vi "open-islanding.vi"(7 "islanding config":T1={"GA-ip"="192.168.1.1", "write-port-ga"=32101, "listen-port"=32111, "res-ip"="127.0.0.1", "write-port-res"=32102}) -> (0 "error out":errorcluster, 5 "connection ID":refnum<k16>)   [LabVIEW 2021]
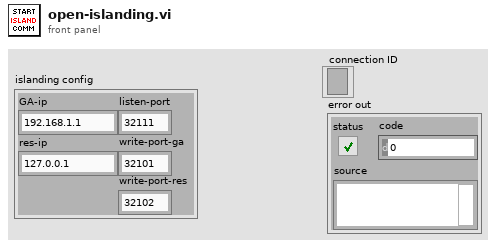
[diagram p1: front panel]
types:
  T1 = cluster{"GA-ip":string, "write-port-ga":u16, "listen-port":u16, "res-ip":string, "write-port-res":u16}
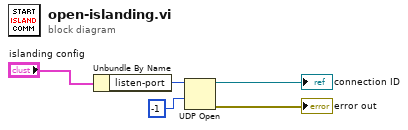
[diagram p0: block diagram]
diagram:
  n1 = Unbundle By Name("islanding config") -> ("listen-port"=w3:u16)
  n2 = UDP Open(9:-1 ("timeout ms (25000)"), 11:w3) -> (port=→"connection ID":refnum<k16>, 0:→"error out":errorcluster)  [unwired: 3 in, 1 out]
